vi "Constructor.vi"(8 "error in (no error)":errorcluster, 10 "Init Command":string, 11 "VISA resource name":refnum<visa-resource-name>) -> (0 "error out":errorcluster, 3 "LED Matrix out":refnum<class "LED Matrix.lvclass">)   [LabVIEW 2026, in "LED Matrix.lvlib" / "LED Matrix.lvclass"]
uses:
  LED Matrix.lvclass
  LED Matrix.lvclass/LED Matrix.ctl
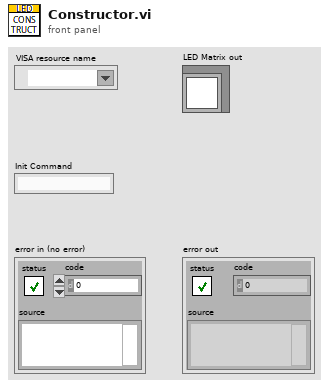
[diagram p1: front panel]
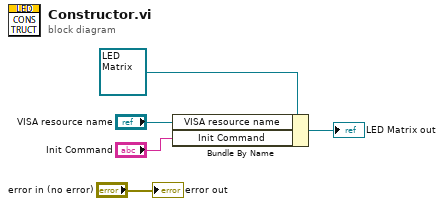
[diagram p0: block diagram]
diagram:
  n1 = Bundle By Name(cluster=refnum<class "LED Matrix.lvclass"> refnum ("LED Matrix in"), "VISA resource name"="VISA resource name", "Init Command"="Init Command") -> (→"LED Matrix out":refnum<class "LED Matrix.lvclass">)
  "error out" <- "error in (no error)"
